vi "ComputeIndentation.vi"(11 "MsgSerializer in":refnum<class "MsgSerializer.JSON.lvclass">) -> (2 "indentation":string)   [LabVIEW 2020]
uses:
  MsgSerializer.JSON.lvclass
  C:/projects/caraya/src/classes/MsgSerializer/MsgSerializer.lvclass
  C:/projects/caraya/src/classes/MsgSerializer.JSON/MsgSerializer/MsgSerializer.JSON.lvclass
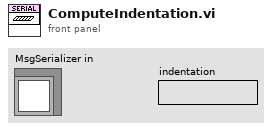
[diagram p1: front panel]
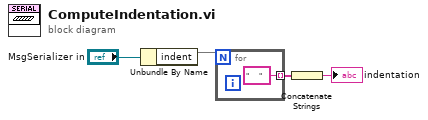
[diagram p0: block diagram]
diagram:
  n1 = Unbundle By Name("MsgSerializer in") -> ("indent"=w2)
  n2 = for {
    N: w2 -> [_]
    tunnel: ["     " ("string")] -> w3 mode=indexing
  }
  n3 = Concatenate Strings(w3) -> (→"indentation":string)
